vi "get_component_readiness.vi"(8 "error in (no error)":errorcluster, 10 "top-level components":T1[](array[typedef]), 11 "control references":T2) -> (0 "error out":errorcluster, 2 "ready?":bool)   [LabVIEW 2010]
uses:
  type_definitions/clusters/controls_refs.ctl
  common/enumerations/top-level_component_type_enum.ctl
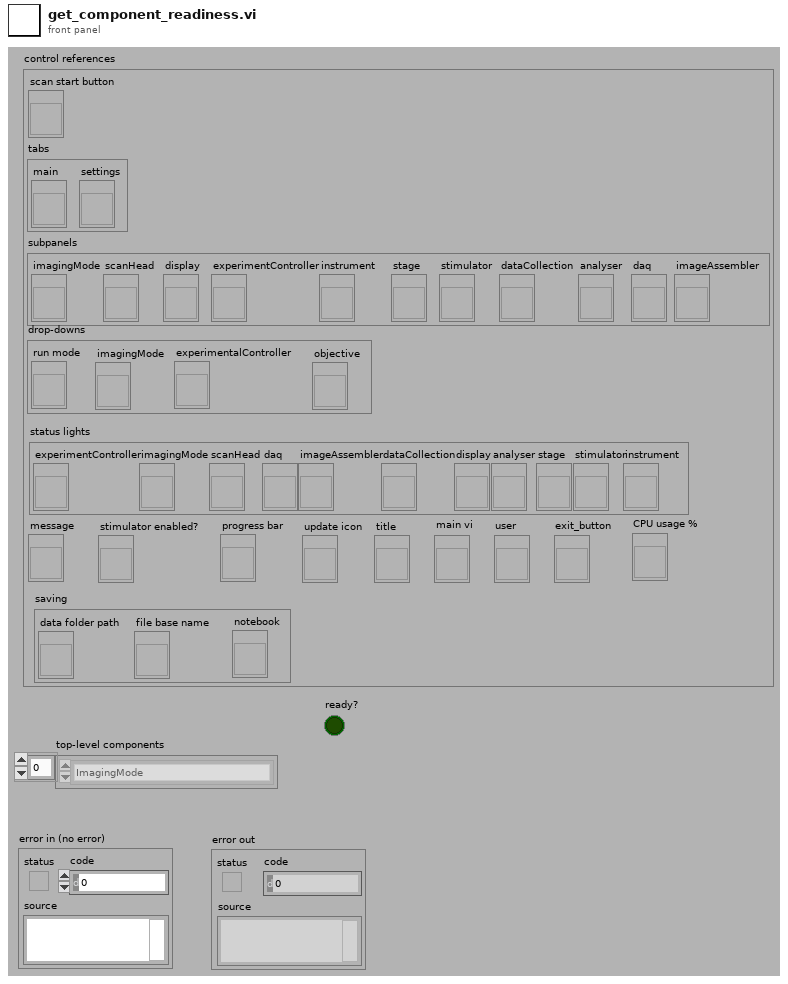
[diagram p1: front panel]
types:
  T1 = typedef "top-level_component_type_enum.ctl" = enum16{"ImagingMode", "ScanHead", "DAQ", "ImageAssembler", "Display", "DataCollection", "Analyser", "Stimulator", "ExperimentController", "Instrument", "Stage"}
  T2 = typedef "controls_refs.ctl" = cluster{"scan start button":refnum<vi>, "tabs":cluster{"main":refnum<vi>, "settings":refnum<vi>}, "subpanels":cluster{"imagingMode":refnum<vi>, "scanHead":refnum<vi>, "display":refnum<vi>, "experimentController":refnum<vi>, "instrument":refnum<vi>, "stage":refnum<vi>, "stimulator":refnum<vi>, "dataCollection":refnum<vi>, "analyser":refnum<vi>, "daq":refnum<vi>, "imageAssembler":refnum<vi>}, "drop-downs":cluster{"run mode":refnum<vi>, "imagingMode":refnum<vi>, "experimentalController":refnum<vi>, "objective":refnum<vi>}, "status lights":cluster{"experimentController":refnum<vi>, "imagingMode":refnum<vi>, "scanHead":refnum<vi>, "daq":refnum<vi>, "imageAssembler":refnum<vi>, "dataCollection":refnum<vi>, "display":refnum<vi>, "analyser":refnum<vi>, "stage":refnum<vi>, "stimulator":refnum<vi>, "instrument":refnum<vi>}, "message":refnum<vi>, "stimulator enabled?":refnum<vi>, "saving":cluster{"data folder path":refnum<vi>, "file base name":refnum<vi>, "notebook":refnum<vi>}, "progress bar":refnum<vi>, "update icon":refnum<vi>, "title":refnum<vi>, "main vi":refnum<vi>, "user":refnum<vi>, "exit_button":refnum<vi>, "CPU usage %":refnum<vi>}
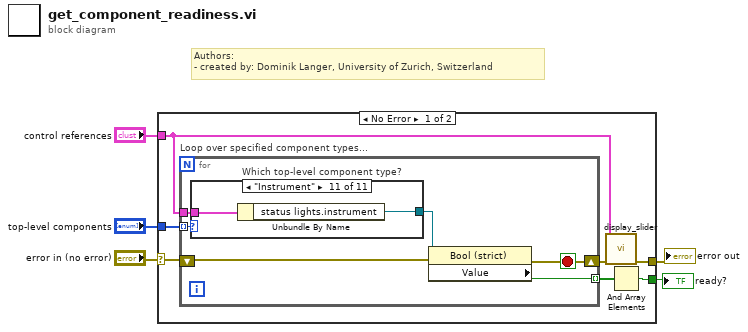
[diagram p0: block diagram]
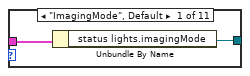
[diagram p2: hidden frame]
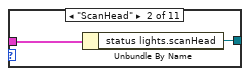
[diagram p3: hidden frame]
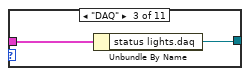
[diagram p4: hidden frame]
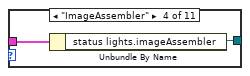
[diagram p5: hidden frame]
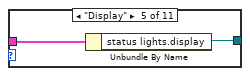
[diagram p6: hidden frame]
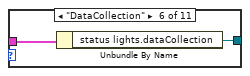
[diagram p7: hidden frame]
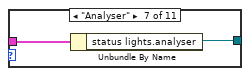
[diagram p8: hidden frame]
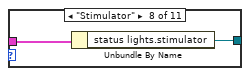
[diagram p9: hidden frame]
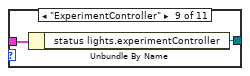
[diagram p10: hidden frame]
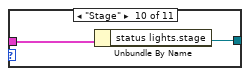
[diagram p11: hidden frame]
diagram:
  # "Authors: \n- created by: Dominik Langer, University of Zurich, Switzerland"
  n1 = case shown="No Error" "error in (no error)" {
    selector: "error in (no error)" -> [w11 w41]
    tunnel: "control references" -> [w10 _]
    tunnel: [w9 w41] -> w2
    tunnel: "top-level components" -> [w8 _]
    tunnel: [w7 _] -> w5
    frame No Error {
      n2 = for "Loop over specified component types..." {
        tunnel: w10 -> [w17]
        tunnel: w8 -> [w15] mode=indexing
        tunnel: [w14] -> w6 mode=indexing
        shift-right: [w13] -> w12
        shift-left: w11 -> [w18]
        stop <- w13 stop-if-true
        n3 = case "Which top-level component type?" shown="\"Instrument\"" w15 {
          tunnel: w17 -> [w20 w22 w24 w26 w28 w30 w32 w34 w36 w37 w40]
          tunnel: [w19 w21 w23 w25 w27 w29 w31 w33 w35 w38 w39] -> w16
          frame "ImagingMode", Default {
            n4 = Unbundle By Name(w20) -> ("status lights.imagingMode"=w19:refnum<vi>)
          }
          frame "ScanHead" {
            n5 = Unbundle By Name(w22) -> ("status lights.scanHead"=w21:refnum<vi>)
          }
          frame "DAQ" {
            n6 = Unbundle By Name(w24) -> ("status lights.daq"=w23:refnum<vi>)
          }
          frame "ImageAssembler" {
            n7 = Unbundle By Name(w26) -> ("status lights.imageAssembler"=w25:refnum<vi>)
          }
          frame "Display" {
            n8 = Unbundle By Name(w28) -> ("status lights.display"=w27:refnum<vi>)
          }
          frame "DataCollection" {
            n9 = Unbundle By Name(w30) -> ("status lights.dataCollection"=w29:refnum<vi>)
          }
          frame "Analyser" {
            n10 = Unbundle By Name(w32) -> ("status lights.analyser"=w31:refnum<vi>)
          }
          frame "Stimulator" {
            n11 = Unbundle By Name(w34) -> ("status lights.stimulator"=w33:refnum<vi>)
          }
          frame "ExperimentController" {
            n12 = Unbundle By Name(w36) -> ("status lights.experimentController"=w35:refnum<vi>)
          }
          frame "Stage" {
            n13 = Unbundle By Name(w37) -> ("status lights.stage"=w38:refnum<vi>)
          }
          frame "Instrument" {
            n14 = Unbundle By Name(w40) -> ("status lights.instrument"=w39:refnum<vi>)
          }
        }
        n15 = property class="Bool (strict)"(reference=w16, error in=w18) -> (error out=w13:errorcluster, "Value"=w14:bool)  [unwired: 1 out]
      }
      n16 = call "display_slider.vi"("error in"=w12, "cluster refs in"=w10) -> ("error out"=w9:errorcluster)  [unwired: 9 in]
      n17 = And Array Elements(Boolean array=w6) -> (logical AND=w7:bool)
    }
    frame Error {
    }
  }
  "error out" <- w2
  "ready?" <- w5
